vi "USBCLIENT2.vi"() -> ()   [LabVIEW 2018]
uses:
  <vilib>/daq.io/MQTT LabVIEW Client/Controls/QoS.ctl
  <vilib>/daq.io/MQTT LabVIEW Client/Controls/DUP_Flag.ctl
  <vilib>/daq.io/MQTT LabVIEW Client/Controls/Retain_Flag.ctl
  <vilib>/daq.io/MQTT LabVIEW Client/Controls/Connect_Flags.ctl
  <vilib>/daq.io/MQTT LabVIEW Client/Controls/User_Info.ctl
  <vilib>/DAQmx/read.llb/DAQmx Read (Analog DBL 1Chan 1Samp).vi
  <vilib>/DAQmx/write.llb/DAQmx Write (Analog DBL 1Chan 1Samp).vi
  <vilib>/DAQmx/create/channels.llb/DAQmx Create Channel (AI-Voltage-Basic).vi
  <vilib>/DAQmx/create/channels.llb/DAQmx Create Channel (AO-Voltage-Basic).vi
  <vilib>/DAQmx/miscellaneous.llb/DAQmx Fill In Error Info.vi
  <vilib>/daq.io/MQTT LabVIEW Client/MQTT_Functions.lvlib
panel:
  in  "stop":bool
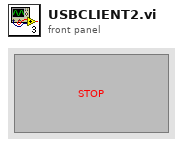
[diagram p1: front panel]
types:
  T1 = typedef "MQTT_Functions.lvlib/User_Info.ctl" = cluster{"User Name":string, "Password":string}
  T2 = typedef "MQTT_Functions.lvlib/QoS.ctl" = enum8{"At most once", "At least once", "Exactly once", "Reserved"}
  T3 = typedef "MQTT_Functions.lvlib/Connect_Flags.ctl" = cluster{"user name":bool, "password":bool, "will retain":bool, "will flag":bool, "clean session":bool, "reserved":bool, "will QoS":T2}
  T4 = typedef "MQTT_Functions.lvlib/DUP_Flag.ctl" = bool
  T5 = typedef "MQTT_Functions.lvlib/Retain_Flag.ctl" = bool
  T6 = cluster{"QoS":T2, "DUP":T4, "Retain":T5, "Keep Alive (sec)":u16}
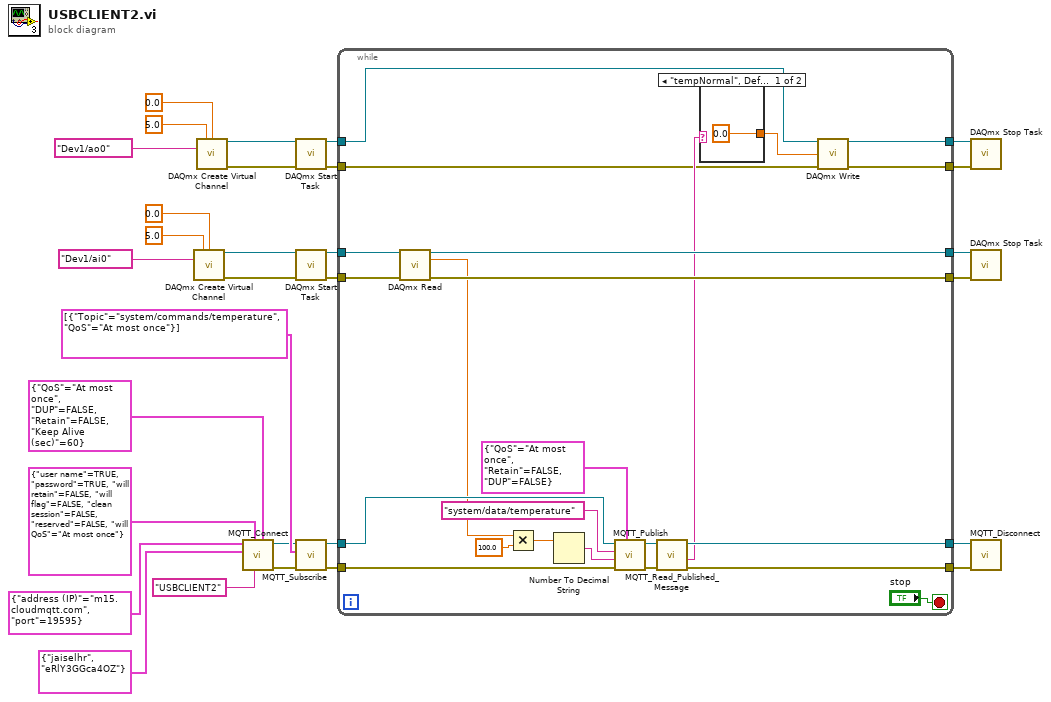
[diagram p0: block diagram]
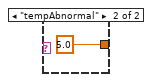
[diagram p2: hidden frame]
diagram:
  n1 = call-poly <vilib>:"DAQmx Create Virtual Channel.vi"("maximum value"=5.0, "minimum value"=0.0, "physical channels"=tag "Dev1/ai0") -> ("task out"=w18:refnum<k21>, "error out"=w17:errorcluster)  [unwired: 11 in]
  n2 = call-poly <vilib>:"DAQmx Create Virtual Channel.vi"("maximum value"=5.0, "minimum value"=0.0, "physical channels"=tag "Dev1/ao0") -> ("task out"=w6:refnum<k21>, "error out"=w5:errorcluster)  [unwired: 11 in]
  n3 = call <vilib>:"MQTT_Connect.vi"("Connect Meta"=T6 {"QoS"=enum."At most once", "DUP"=FALSE, "Retain"=FALSE, "Keep Alive (sec)"=60}, "Client ID"="USBCLIENT2", "Connect Flags"=T3 {"user name"=TRUE, "password"=TRUE, "will retain"=FALSE, "will flag"=FALSE, "clean session"=FALSE, "reserved"=FALSE, "will QoS"=enum."At most once"}, "User Info"=T1 {"User Name"="jaiselhr", "Password"="eRlY3GGca4OZ"}, "MQTT Broker"=cluster{"address (IP)":string, "port":u16} {"address (IP)"="m15.cloudmqtt.com", "port"=19595}) -> ("error out"=w24:errorcluster, "connection ID out"=w22:refnum<k5>)  [unwired: 4 in, 1 out]
  n4 = call <vilib>:"DAQmx Start Task.vi"("task/channels in"=w6, "error in"=w5) -> ("task out"=w10:refnum<k21>, "error out"=w9:errorcluster)  [unwired: 12 in]
  n5 = call <vilib>:"DAQmx Start Task.vi"("task/channels in"=w18, "error in"=w17) -> ("task out"=w14:refnum<k21>, "error out"=w13:errorcluster)  [unwired: 12 in]
  n6 = call <vilib>:"MQTT_Subscribe.vi"("error in (no error)"=w24, "Subscription Info Array"=cluster{"Topic":string, "QoS":T2}[] [{"Topic"="system/commands/temperature", "QoS"=enum."At most once"}], "connection ID"=w22) -> ("error out"=w21:errorcluster, "connection ID out"=w20:refnum<k5>)  [unwired: 7 in]
  n7 = while {
    tunnel: [w51] -> w26
    tunnel: [w50] -> w25
    tunnel: w21 -> [w49]
    tunnel: w20 -> [w48]
    tunnel: w14 -> [w46]
    tunnel: w13 -> [w45]
    tunnel: [w44] -> w12
    tunnel: [w43] -> w11
    tunnel: w10 -> [w39]
    tunnel: w9 -> [w38]
    tunnel: [w37] -> w8
    tunnel: [w36] -> w7
    stop <- "stop" stop-if-true
    n8 = call-poly <vilib>:"DAQmx Read.vi"("task/channels in"=w46, "error in"=w45) -> ("task out"=w44:refnum<k21>, "data"=w33:dbl, "error out"=w43:errorcluster)  [unwired: 11 in]
    n9 = Multiply(x=w33, y=100.0) -> (x*y=w31:dbl)
    n10 = Number To Decimal String(number=w31) -> (decimal integer string=w35:string)  [unwired: 1 in]
    n11 = call <vilib>:"MQTT_Publish.vi"("Publish Meta"=cluster{"QoS":T2, "Retain":T5, "DUP":T4} {"QoS"=enum."At most once", "Retain"=FALSE, "DUP"=FALSE}, "error in (no error)"=w49, "Message to be published"=w35, "Topic"="system/data/temperature", "connection ID"=w48) -> ("error out"=w53:errorcluster, "connection ID out"=w52:refnum<k5>)  [unwired: 5 in]
    n12 = call <vilib>:"MQTT_Read_Published_Message.vi"("error in (no error)"=w53, "connection ID"=w52) -> ("error out"=w51:errorcluster, "Message"=w40:string, "connection ID out"=w50:refnum<k5>)  [unwired: 4 in, 3 out]
    n13 = case shown="\"tempNormal\", Default" w40 {
      tunnel: [0.0 ("data") 5.0 ("data")] -> w34
      frame "tempNormal", Default {
      }
      frame "tempAbnormal" {
      }
    }
    n14 = call-poly <vilib>:"DAQmx Write.vi"("task/channels in"=w39, "data"=w34, "error in"=w38) -> ("task out"=w37:refnum<k21>, "error out"=w36:errorcluster)  [unwired: 10 in, 1 out]
  }
  n15 = call <vilib>:"DAQmx Stop Task.vi"("task/channels in"=w8, "error in"=w7) -> ()  [unwired: 12 in, 2 out]
  n16 = call <vilib>:"DAQmx Stop Task.vi"("task/channels in"=w12, "error in"=w11) -> ()  [unwired: 12 in, 2 out]
  n17 = call <vilib>:"MQTT_Disconnect.vi"("error in (no error)"=w26, "connection ID"=w25) -> ()  [unwired: 9 in, 1 out]
